vi "Main.vi"() -> ()   [LabVIEW 2019]
uses:
  Controles/Slide.ctl
panel:
  in  "generarC1":bool
  in  "Vertical Pointer Slide":T1 scale=0.0..10.0
  out "voltMonA_2":dbl format="%.1f"
  out "frecMonA_2":dbl format="%.1f"
  # "Monitoreo"
  # "Frecuencia"
  # "Hz"
  # "Voltaje"
  # "mV"
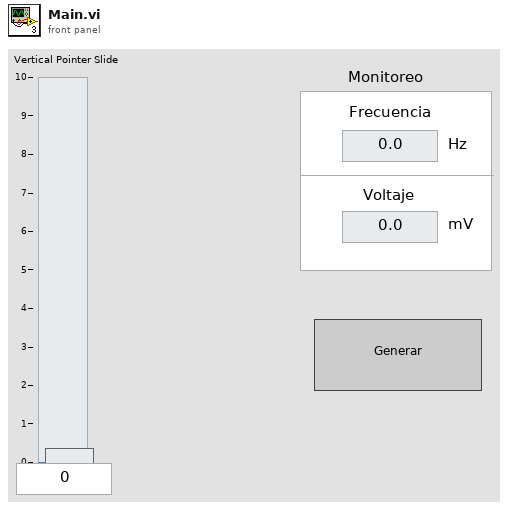
[diagram p1: front panel]
types:
  T1 = typedef "Slide.ctl" = dbl
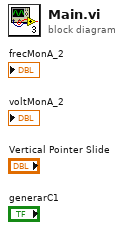
[diagram p0: block diagram]
diagram:
